vi "UpdateListMenu.vi"(0 "ListBox in":refnum<vi>, 1 "MenuRef":refnum<k9>, 2 "PointedRow":i32) -> ()   [LabVIEW 2017, in "XListGraph.lvlib" / "XListGraph.xctl"]
uses:
  XListGraph.xctl
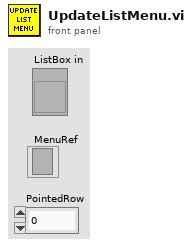
[diagram p1: front panel]
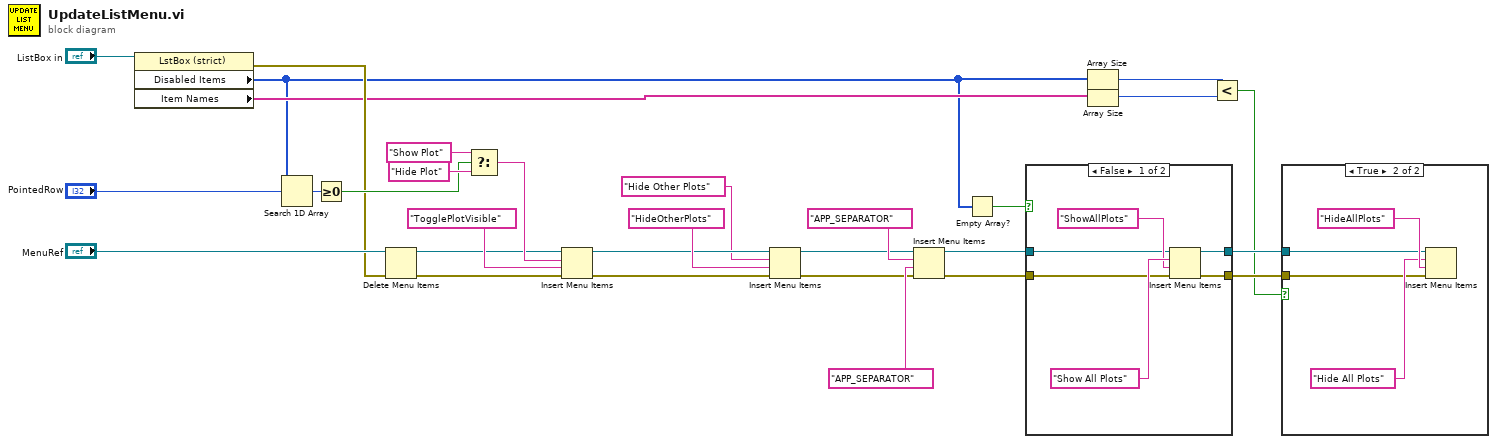
[diagram p0: block diagram]
diagram:
  n1 = property class="LstBox (strict)"(reference="ListBox in") -> (error out=w20:errorcluster, "Disabled Items"=w10:i32[], "Item Names"=w11:string[])  [unwired: 1 in, 1 out]
  n2 = Search 1D Array(1D array=w10, element="PointedRow") -> (index of element=w27:i32)  [unwired: 1 in]
  n3 = Greater Or Equal To 0?(x=w27) -> (x >= 0?=w24:bool)
  n4 = Delete Menu Items(6:w20, 9:"MenuRef") -> (0:w19:errorcluster, 3:w21:refnum<k9>)  [unwired: 2 in]
  n5 = Select(t="Show Plot", s=w24, f="Hide Plot") -> (s? t:f=w23:string)
  n6 = Insert Menu Items(6:w19, 7:"TogglePlotVisible" ("item names"), 8:w23, 9:w21) -> (0:w5:errorcluster, 3:w4:refnum<k9>)  [unwired: 2 in, 1 out]
  n7 = Insert Menu Items(6:w5, 7:"HideOtherPlots" ("item names"), 8:"Hide Other Plots" ("item names"), 9:w4) -> (0:w2:errorcluster, 3:w3:refnum<k9>)  [unwired: 2 in, 1 out]
  n8 = Insert Menu Items(6:w2, 7:"APP_SEPARATOR", 8:"APP_SEPARATOR" ("item names"), 9:w3) -> (0:w15:errorcluster, 3:w16:refnum<k9>)  [unwired: 2 in, 1 out]
  n9 = Empty Array?(array=w10) -> (empty?=w12:bool)
  n10 = case shown="False" w12 {
    tunnel: [w34 w38] -> w18
    tunnel: [w33 w37] -> w17
    tunnel: w16 -> [w32 w38]
    tunnel: w15 -> [w31 w37]
    frame False {
      n11 = Insert Menu Items(6:w31, 7:"ShowAllPlots" ("item names"), 8:"Show All Plots", 9:w32) -> (0:w33:errorcluster, 3:w34:refnum<k9>)  [unwired: 2 in, 1 out]
    }
    frame True {
    }
  }
  n12 = Array Size(array=w10) -> (size(s)=w9:i32)
  n13 = Array Size(array=w11) -> (size(s)=w8:i32)
  n14 = Less?(x=w9, y=w8) -> (x < y?=w7:bool)
  n15 = case shown="True" w7 {
    tunnel: w18 -> [_ w40]
    tunnel: w17 -> [_ w39]
    frame False {
    }
    frame True {
      n16 = Insert Menu Items(6:w39, 7:"HideAllPlots" ("item names"), 8:"Hide All Plots", 9:w40) -> ()  [unwired: 2 in, 3 out]
    }
  }
